vi "SetDelay.vi"(2 "Digitizer delay\n (ms)":dbl format="%.2f", 3 "Delay Mod (micsec)":dbl format="%.3f") -> (0 "error out":errorcluster, 1 "ActXDSO":refnum<k7>)   [LabVIEW 2022 SP3]
uses:
  Motion Controllers/-MotionRoutines/MotionGlobals.vi
panel:
  in  "error in":errorcluster
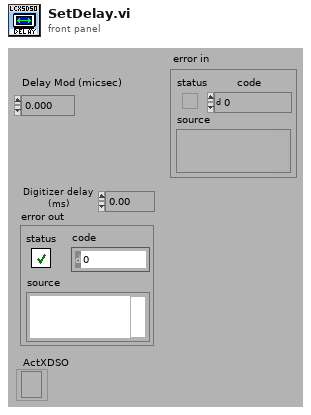
[diagram p1: front panel]
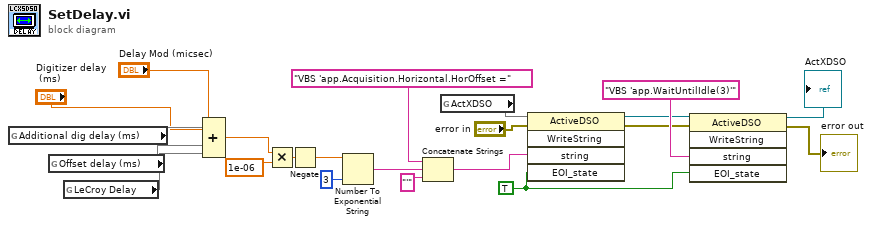
[diagram p0: block diagram]
diagram:
  w5 = TRUE
  n1 = global read "MotionGlobals.vi" "Additional dig delay (ms)"() -> (w22)
  n2 = global read "MotionGlobals.vi" "Offset delay (ms)"() -> (w21)
  n3 = global read "MotionGlobals.vi" "LeCroy Delay"() -> (w20)
  n4 = Compound Arithmetic op=ADD("Delay Mod (micsec)", "Digitizer delay\n (ms)", w22, w21, w20) -> (w12:dbl)
  n5 = Multiply(x=w12, y=1e-06) -> (x*y=w11:dbl)
  n6 = Negate(x=w11) -> (-x=w14:dbl)
  n7 = Number To Exponential String(number=w14, precision (6)=3) -> (E-format string=w16:string)  [unwired: 2 out]
  n8 = Concatenate Strings("VBS 'app.Acquisition.Horizontal.HorOffset =", w16, "'") -> (w10:string)
  n9 = global read "MotionGlobals.vi" "ActXDSO"() -> (w9)
  n10 = invoke class="ActiveDSO" method="WriteString"(reference=w9, error in="error in", "string"=w10, "EOI_state"=w5) -> (reference out=w7:refnum<k7>, error out=w6:errorcluster)  [unwired: 1 in, 3 out]
  n11 = invoke class="ActiveDSO" method="WriteString"(reference=w7, error in=w6, "string"="VBS 'app.WaitUntilIdle(3)'", "EOI_state"=w5) -> (reference out=→"ActXDSO":refnum<k7>, error out=→"error out":errorcluster)  [unwired: 1 in, 3 out]
